vi "Path for initialisation file.vi"(9 "Init File Name":string, 11 "VI Path":path) -> (3 "Required Path":path)   [LabVIEW 2011]
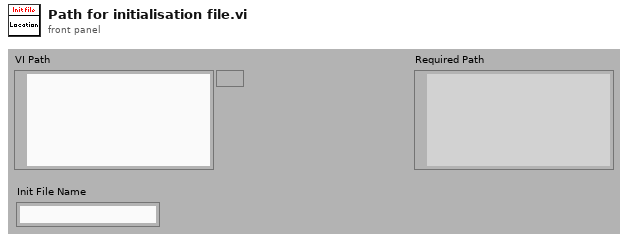
[diagram p1: front panel]
types:
  T1 = enum32{"invalid app kind", "Development System", "Run Time System", "Student Edition", "Embedded LabVIEW", "Evaluation", "Custom"}
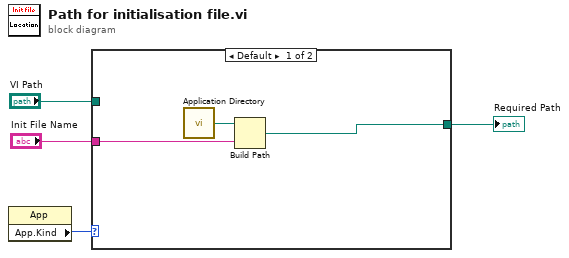
[diagram p0: block diagram]
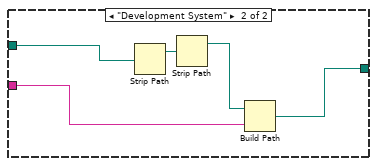
[diagram p2: hidden frame]
diagram:
  n1 = property class="App"() -> ("App.Kind"=w4:T1)  [unwired: 2 in, 2 out]
  n2 = case shown="Default" w4 {
    tunnel: "VI Path" -> [_ w11]
    tunnel: "Init File Name" -> [w6 w9]
    tunnel: [w5 w8] -> w1
    frame Default {
      n3 = call <vilib>:"Application Directory.vi"() -> ("Application Directory"=w7:path)
      n4 = Build Path(base path=w7, name or relative path=w6) -> (appended path=w5:path)
    }
    frame "Development System" {
      n5 = Strip Path(path=w11) -> (stripped path=w12:path)  [unwired: 1 out]
      n6 = Strip Path(path=w12) -> (stripped path=w10:path)  [unwired: 1 out]
      n7 = Build Path(base path=w10, name or relative path=w9) -> (appended path=w8:path)
    }
  }
  "Required Path" <- w1
